vi "file_path.vi"(10 "name identifier":string, 11 "Base path":path=path "C:/Users/MPI/Desktop") -> (0 "HDF path":path, 1 "TDMS path":path)   [LabVIEW 2019]
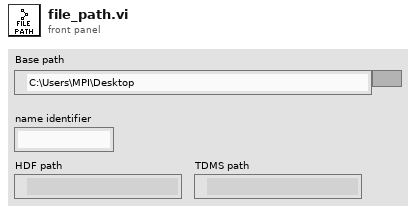
[diagram p1: front panel]
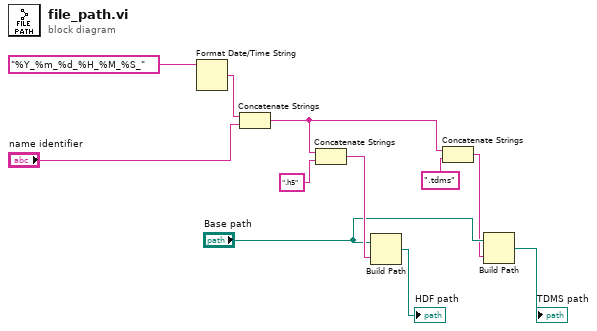
[diagram p0: block diagram]
diagram:
  n1 = Format Date/Time String(time format string (%c)="%Y_%m_%d_%H_%M_%S_") -> (date/time string=w11:string)  [unwired: 2 in]
  n2 = Concatenate Strings(w11, "name identifier") -> (w7:string)
  n3 = Concatenate Strings(w7, ".h5" ("string")) -> (w6:string)
  n4 = Build Path(base path="Base path", name or relative path=w6) -> (appended path=→"HDF path":path)
  n5 = Concatenate Strings(w7, ".tdms" ("string")) -> (w3:string)
  n6 = Build Path(base path="Base path", name or relative path=w3) -> (appended path=→"TDMS path":path)
